vi "CRYGet Access Level Message.vi"(11 "sAction":string) -> (3 "Multibyte string":string)   [LabVIEW 2013]
uses:
  CRYMainGlobal.vi
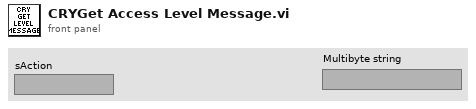
[diagram p1: front panel]
types:
  T1 = enum32{"English", "Chinese", "Korean", "Japanese", "Russian", "Chinese traditional"}
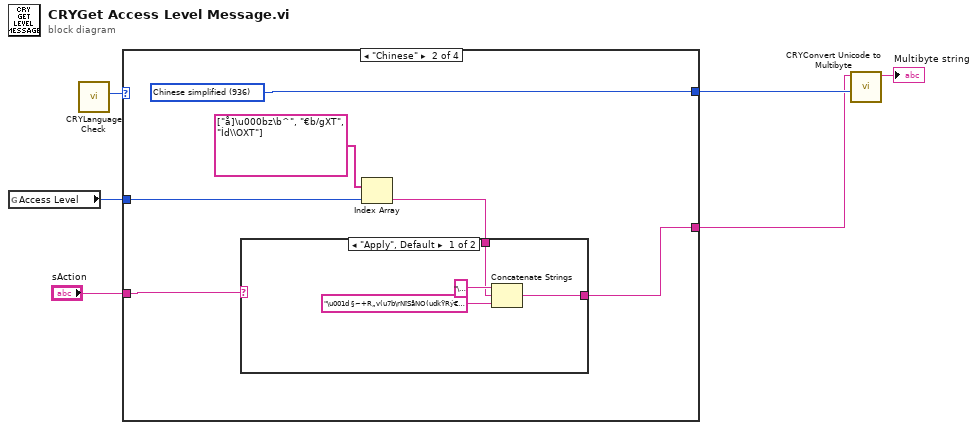
[diagram p0: block diagram]
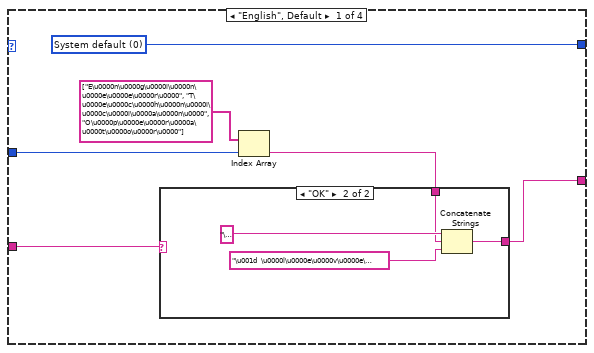
[diagram p2: hidden frame]
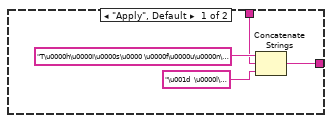
[diagram p3: hidden frame]
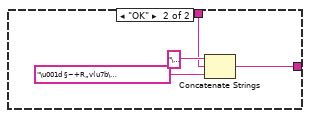
[diagram p4: hidden frame]
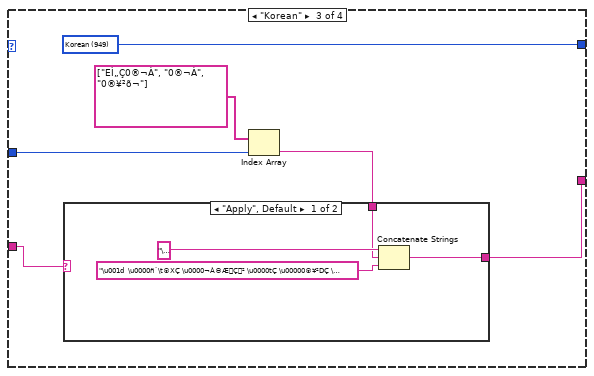
[diagram p5: hidden frame]
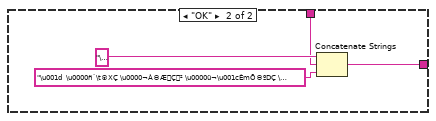
[diagram p6: hidden frame]
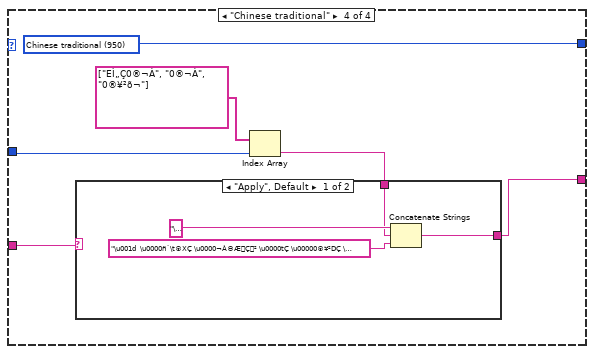
[diagram p7: hidden frame]
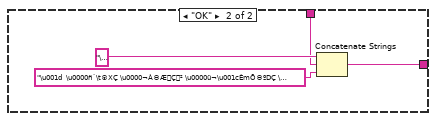
[diagram p8: hidden frame]
diagram:
  n1 = global read "CRYMainGlobal.vi" "Access Level"() -> (w4:enum16{"Engineer", "Technician", "Operator"})
  n2 = call "CRYLanguage Check.vi"() -> ("Language"=w6:T1)  [unwired: 10 in, 1 out]
  n3 = case shown="\"Chinese\"" w6 {
    tunnel: [w12 w26 w40 w54] -> w5
    tunnel: w4 -> [w10 w23 w37 w52]
    tunnel: [w9 w22 w36 w50] -> w3
    tunnel: "sAction" -> [w7 w21 w35 w49]
    frame "English", Default {
      w12 = 0 items=["System default"=0, "Latin-1"=1252, "Japanese"=932, "Korean"=947, "Chinese simplified"=936, "Chinese traditional"=950, "Central Europe"=1250, "Cyrillic"=1251, "Greek"=1253, "Turkish"=1254, "Hebrew"=1255, "Arabic"=1256, "Baltic"=1257, "Thai"=874, "Vietnamese"=783, "UTF8"=65001, "UTF-7"=65000] ("Code Page")
      n4 = Index Array(array=string[] ["E\u0000n\u0000g\u0000i\u0000n\u0000e\u0000e\u0000r\u0000", "T\u0000e\u0000c\u0000h\u0000n\u0000i\u0000c\u0000i\u0000a\u0000n\u0000", "O\u0000p\u0000e\u0000r\u0000a\u0000t\u0000o\u0000r\u0000"], index=w10) -> (element=w8:string)
      n5 = case shown="\"OK\"" w7 {
        tunnel: [w14 w18] -> w9
        tunnel: w8 -> [w13 w17]
        frame "Apply", Default {
          n6 = Concatenate Strings("T\u0000h\u0000i\u0000s\u0000 \u0000f\u0000u\u0000n\u0000c\u0000t\u0000i\u0000o\u0000n\u0000 \u0000i\u0000s\u0000 \u0000n\u0000o\u0000t\u0000 \u0000a\u0000c\u0000c\u0000e\u0000s\u0000s\u0000i\u0000b\u0000l\u0000e\u0000 \u0000t\u0000o\u0000 \u0000a\u0000 \u0000\u001d " ("Label.Text"), w13, "\u001d  \u0000l\u0000e\u0000v\u0000e\u0000l\u0000 \u0000u\u0000s\u0000e\u0000r\u0000.\u0000" ("Label.Text")) -> (w14:string)
        }
        frame "OK" {
          n7 = Concatenate Strings("\u001d " ("Label.Text"), w17, "\u001d  \u0000l\u0000e\u0000v\u0000e\u0000l\u0000 \u0000u\u0000s\u0000e\u0000r\u0000 \u0000c\u0000a\u0000n\u0000n\u0000o\u0000t\u0000 \u0000s\u0000a\u0000v\u0000e\u0000 \u0000S\u0000t\u0000e\u0000p\u0000.\u0000" ("Label.Text")) -> (w18:string)
        }
      }
    }
    frame "Chinese" {
      w26 = 936 items=["System default"=0, "Latin-1"=1252, "Japanese"=932, "Korean"=947, "Chinese simplified"=936, "Chinese traditional"=950, "Central Europe"=1250, "Cyrillic"=1251, "Greek"=1253, "Turkish"=1254, "Hebrew"=1255, "Arabic"=1256, "Baltic"=1257, "Thai"=874, "Vietnamese"=783, "UTF8"=65001, "UTF-7"=65000] ("Code Page")
      n8 = Index Array(array=string[] ["å]\u000bz\b^", "€b/gXT", "Íd\\OXT"], index=w23) -> (element=w25:string)
      n9 = case shown="\"Apply\", Default" w21 {
        tunnel: w25 -> [w29 w33]
        tunnel: [w27 w31] -> w22
        frame "Apply", Default {
          n10 = Concatenate Strings("\u001d " ("Label.Text"), w29, "\u001d §~+R„v(u7b\rNïSåNO(udkŸRý€.\u0000" ("Label.Text")) -> (w27:string)
        }
        frame "OK" {
          n11 = Concatenate Strings("\u001d " ("Label.Text"), w33, "\u001d §~+R„v(u7b\rNïSåNÝOX[ek¤š.\u0000" ("Label.Text")) -> (w31:string)
        }
      }
    }
    frame "Korean" {
      w40 = 949 items=["System default"=0, "Latin-1"=1252, "Japanese"=932, "Korean"=949, "Chinese simplified"=936, "Chinese traditional"=950, "Central Europe"=1250, "Cyrillic"=1251, "Greek"=1253, "Turkish"=1254, "Hebrew"=1255, "Arabic"=1256, "Baltic"=1257, "Thai"=874, "Vietnamese"=783, "UTF8"=65001, "UTF-7"=65000] ("Code Page")
      n12 = Index Array(array=string[] ["EÌ„Ç0®¬À", "0®¬À", "0®¥²õ¬"], index=w37) -> (element=w39:string)
      n13 = case shown="\"Apply\", Default" w35 {
        tunnel: w39 -> [w43 w47]
        tunnel: [w41 w45] -> w36
        frame "Apply", Default {
          n14 = Concatenate Strings("\u001d " ("Label.Text"), w43, "\u001d  \u0000ñ´\t®XÇ \u0000¬À©ÆÇ² \u0000tÇ \u00000®¥²DÇ \u0000¬¹©Æ`Õ\u0018Â \u0000ÆÅµÂÈ²ä².\u0000" ("Label.Text")) -> (w41:string)
        }
        frame "OK" {
          n15 = Concatenate Strings("\u001d " ("Label.Text"), w47, "\u001d  \u0000ñ´\t®XÇ \u0000¬À©ÆÇ² \u0000ü¬\u001cÈmÕ©ºDÇ \u0000ô¼\u0000­`Õ\u0018Â \u0000ÆÅµÂÈ²ä².\u0000" ("Label.Text")) -> (w45:string)
        }
      }
    }
    frame "Chinese traditional" {
      w54 = 950 items=["System default"=0, "Latin-1"=1252, "Japanese"=932, "Korean"=949, "Chinese simplified"=936, "Chinese traditional"=950, "Central Europe"=1250, "Cyrillic"=1251, "Greek"=1253, "Turkish"=1254, "Hebrew"=1255, "Arabic"=1256, "Baltic"=1257, "Thai"=874, "Vietnamese"=783, "UTF8"=65001, "UTF-7"=65000] ("Code Page")
      n16 = Index Array(array=string[] ["EÌ„Ç0®¬À", "0®¬À", "0®¥²õ¬"], index=w52) -> (element=w51:string)
      n17 = case shown="\"Apply\", Default" w49 {
        tunnel: w51 -> [w57 w61]
        tunnel: [w55 w59] -> w50
        frame "Apply", Default {
          n18 = Concatenate Strings("\u001d " ("Label.Text"), w57, "\u001d  \u0000ñ´\t®XÇ \u0000¬À©ÆÇ² \u0000tÇ \u00000®¥²DÇ \u0000¬¹©Æ`Õ\u0018Â \u0000ÆÅµÂÈ²ä².\u0000" ("Label.Text")) -> (w55:string)
        }
        frame "OK" {
          n19 = Concatenate Strings("\u001d " ("Label.Text"), w61, "\u001d  \u0000ñ´\t®XÇ \u0000¬À©ÆÇ² \u0000ü¬\u001cÈmÕ©ºDÇ \u0000ô¼\u0000­`Õ\u0018Â \u0000ÆÅµÂÈ²ä².\u0000" ("Label.Text")) -> (w59:string)
        }
      }
    }
  }
  n20 = call "CRYConvert Unicode to Multibyte.vi"("Code Page"=w5, "Unicode String"=w3) -> ("Multibyte string"=→"Multibyte string":string)  [unwired: 8 in, 1 out]
